vi "Cleanup VISA Port.vi"(8 "error in (no error)":errorcluster, 11 "Serial Client in":refnum<class "Serial Client.lvclass">) -> (0 "error out":errorcluster, 3 "Serial Client out":refnum<class "Serial Client.lvclass">)   [LabVIEW 2020, in "Stream-Serial.lvlib" / "Serial Client.lvclass"]
uses:
  Serial Client.lvclass
  Serial Client.lvclass/Serial Client.ctl
  Serial Stream/Serial Stream.lvclass
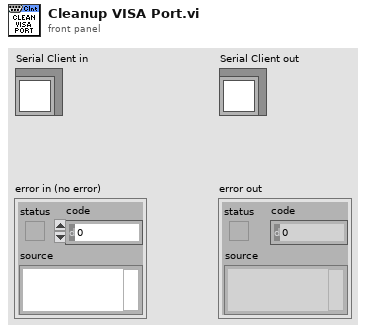
[diagram p1: front panel]
types:
  T1 = typedef "Stream-Serial.lvlib/Serial Client.lvclass/Ref Data.ctl" = cluster{"Stream":refnum<class "Serial Stream.lvclass">, "State":T2, "Client Loop":refnum<vi>, "Port Config":T3}
  T2 = typedef "Stream-Serial.lvlib/Serial Client.lvclass/Connection State.ctl" = enum16{"Closed", "Idle", "Connecting", "Connected", "Shutdown"}
  T3 = typedef "Stream-Serial.lvlib/Serial Client.lvclass/Port Config.ctl" = cluster{"Baud (115200)":u32, "Data Bits (8)":u8, "Stop Bits (1)":T4, "Flow Control":T5, "LineTerm (\\n)":string, "Timeout ms (10000)":i32, "Parity (None)":T6}
  T4 = typedef "Stream-Serial.lvlib/Serial Client.lvclass/Stop Bits.ctl" = u16
  T5 = typedef "Stream-Serial.lvlib/Serial Client.lvclass/Flow Control.ctl" = u16
  T6 = typedef "Stream-Serial.lvlib/Serial Client.lvclass/Parity.ctl" = enum16{"None", "Odd", "Even", "Mark", "Space"}
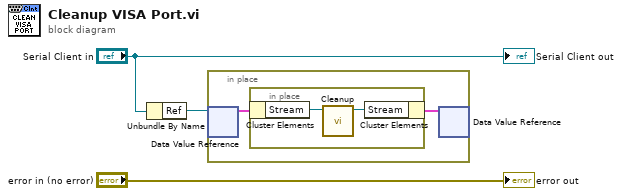
[diagram p0: block diagram]
diagram:
  n1 = Unbundle By Name("Serial Client in") -> ("Ref"=w2:refnum<data-value>)
  n2 = in-place {
    n3 = in-place-dvr #1(w2) -> (w5:T1)  [unwired: 1 out]
    n4 = in-place {
      n5 = in-place-cluster #2(w5) -> ("Stream"=w7:refnum<class "Serial Stream.lvclass">)
      n6 = call "Cleanup.vi"("Serial Stream in"=w7) -> ("Serial Stream out"=w6:refnum<class "Serial Stream.lvclass">)  [unwired: 9 in, 1 out]
      n7 = in-place-cluster #2("Stream"=w6) -> (w4:T1)
    }
    n8 = in-place-dvr #1(w4) -> ()  [unwired: 2 out]
  }
  "error out" <- "error in (no error)"
  "Serial Client out" <- "Serial Client in"
